vi "Get_Connected_with(111)_111_points-1.vi"(7 "[IN] Dot Statuses":i16[][](array[numeric]), 9 "[IN] Indicies of po\nints inside tracks":i32[](array[numeric]), 10 "[IN] Indicies of tracks con\ntaining connected points":i32[](array[numeric])) -> (1 "[OUT] Indicies of tracks co\nntaining connected points":i32[](array[numeric]), 2 "[OUT] Indicies of \npoints inside tracks":i32[](array[numeric]), 3 "[OUT] Candidates for \ncrossconnections are found":bool)   [LabVIEW 2017]
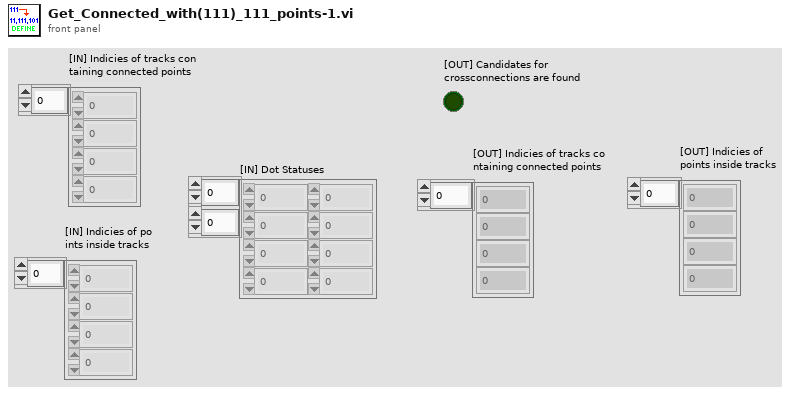
[diagram p1: front panel]
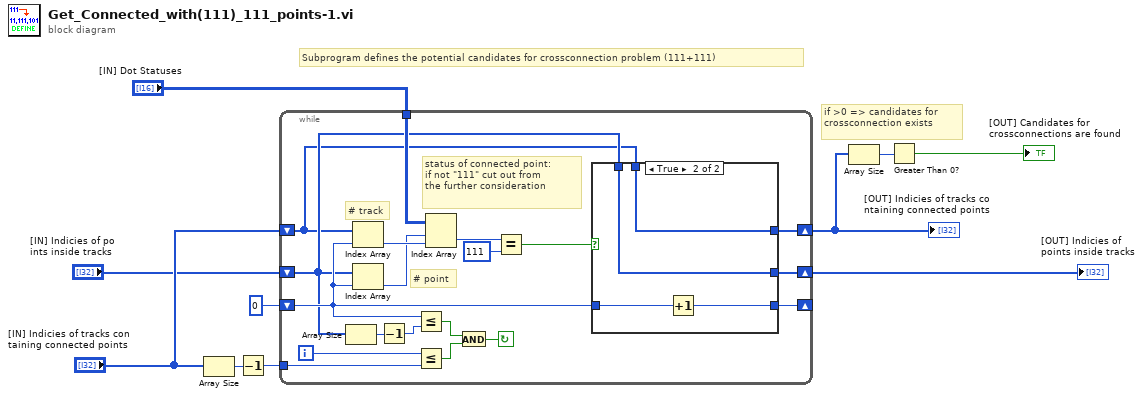
[diagram p0: block diagram]
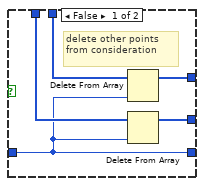
[diagram p2: hidden frame]
diagram:
  # "Subprogram defines the potential candidates for crossconnection problem (111+111)"
  # "if >0 => candidates for\ncrossconnection exists"
  n1 = Array Size(array="[IN] Indicies of tracks con\ntaining connected points") -> (size(s)=w10:i32)
  n2 = Decrement(x=w10) -> (x-1=w9:i32)
  n3 = while {
    tunnel: "[IN] Dot Statuses" -> [w29]
    shift-right: [w14] -> w2
    shift-left: "[IN] Indicies of tracks con\ntaining connected points" -> [w11]
    shift-right: [w13] -> w1
    shift-left: "[IN] Indicies of po\nints inside tracks" -> [w12]
    tunnel: w9 -> [w22]
    shift-right: [w15] -> _
    shift-left: 0 -> [w16]
    i -> [w18]
    stop <- w19 continue-if-true
    # "# point"
    # "# track"
    # "status of connected point: \nif not \"111\" cut out from \nthe further consideration"
    n4 = Array Size(array=w12) -> (size(s)=w24:i32)
    n5 = Index Array(array=w11, index=w16) -> (element=w26:i32)
    n6 = Index Array(array=w12, index=w16) -> (element=w25:i32)
    n7 = Decrement(x=w24) -> (x-1=w23:i32)
    n8 = Less Or Equal?(x=w16, y=w23) -> (x <= y?=w21:bool)
    n9 = Less Or Equal?(x=w18, y=w22) -> (x <= y?=w20:bool)
    n10 = Index Array(array=w29, index (row)=w25, index (col)=w26) -> (element=w27:i16)
    n11 = And(x=w21, y=w20) -> (x .and. y?=w19:bool)
    n12 = Equal?(x=w27, y=i16 111) -> (x = y?=w17:bool)
    n13 = case shown="True" w17 {
      tunnel: w16 -> [w31 w38]
      tunnel: [w31 w37] -> w15
      tunnel: w11 -> [w34 w36]
      tunnel: w12 -> [w32 w35]
      tunnel: [w33 w36] -> w14
      tunnel: [w30 w35] -> w13
      frame False {
        # "delete other points\nfrom consideration"
        n14 = Delete From Array(array=w34, index=w31) -> (array with subset deleted=w33:i32[])  [unwired: 1 in, 1 out]
        n15 = Delete From Array(array=w32, index=w31) -> (array with subset deleted=w30:i32[])  [unwired: 1 in, 1 out]
      }
      frame True {
        n16 = Increment(x=w38) -> (x+1=w37:i32)
      }
    }
  }
  "[OUT] Indicies of \npoints inside tracks" <- w1
  "[OUT] Indicies of tracks co\nntaining connected points" <- w2
  n17 = Array Size(array=w2) -> (size(s)=w7:i32)
  n18 = Greater Than 0?(x=w7) -> (x > 0?=→"[OUT] Candidates for \ncrossconnections are found":bool)
